vi "AlliGator Select Phasor Plot Data to Export Dialog.vi"(8 "error in (no error)":errorcluster) -> (0 "error out":errorcluster, 1 "OK?":bool caption="OK", 2 "Average Plot Data":bool, 3 "Phasor Plot Exported Data":T1)   [LabVIEW 2021, in "AlliGator Phasor Graph.lvlib"]
doc: "Dialog to select which phasor-related parameters to export as ASCII file."
uses:
  AlliGator Phasor Graph.lvlib
  AlliGator Phasor Plot Exported Data Selection.ctl
  GUI/GUI.lvlib
panel:
  in  "Deselect All":bool
  in  "Select All":bool
  in  "Show/Hide SDV":bool caption="Average Plot Data"
  in  "<tau> (amplitude-weighted) SDV":bool caption="<tau>"
  in  "phasor ratio (amplitude-weighted) SDV":bool caption="phasor ratio"
  in  "<tau> (intensity-weighted) SDV":bool caption="<tau>"
  in  "phasor ratio (intensity-weighted) SDV":bool caption="phasor ratio"
  in  "tau m SDV":bool caption="tau m"
  in  "tau phi SDV":bool caption="tau phi"
  in  "m SDV":bool caption="phi"
  in  "phi SDV":bool caption="m"
  in  "s SDV":bool caption="s"
  in  "g SDV":bool caption="g"
  in  "<tau> (amplitude-weighted)":bool caption="<tau>"
  in  "phasor ratio (amplitude-weighted)":bool caption="phasor ratio"
  in  "y":bool caption="s"
  in  "x":bool caption="g"
  in  "<tau> (intensity-weighted)":bool caption="<tau>"
  in  "phasor ratio (intensity-weighted)":bool caption="phasor ratio"
  in  "tau m":bool
  in  "tau phi":bool
  in  "m":bool caption="phi"
  in  "phi":bool caption="m"
  in  "s":bool
  in  "g":bool
  in  "Average Plot Data":bool
  in  "Cancel":bool
  in  "OK":bool caption="OK2"
  # "Select Phasor Plot Data to Export:"
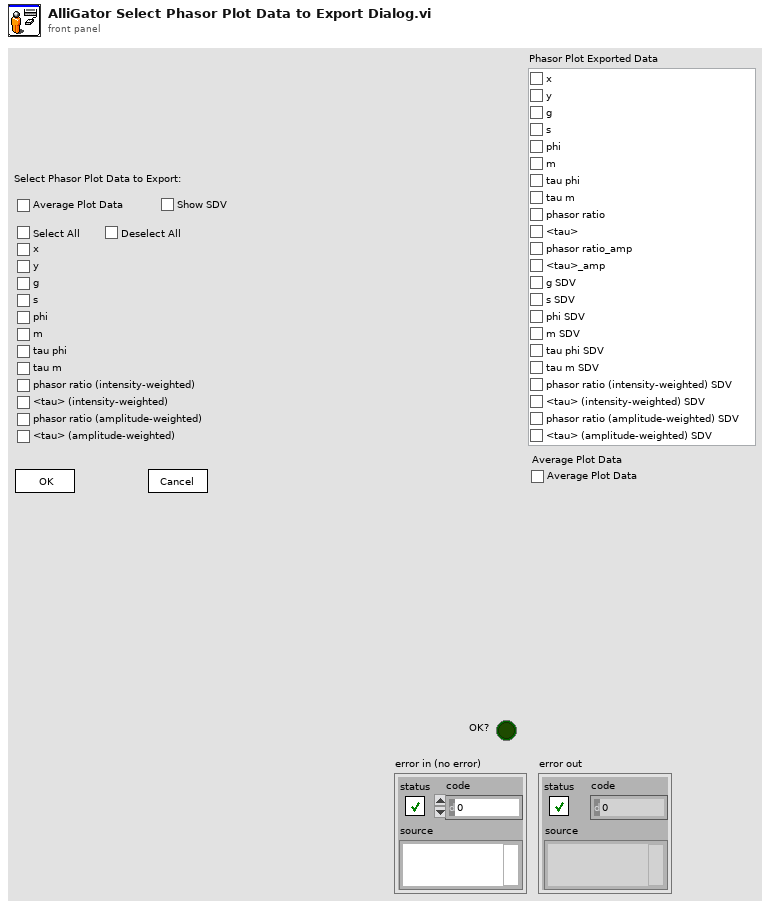
[diagram p1: front panel]
types:
  T1 = typedef "AlliGator Phasor Graph.lvlib/AlliGator Phasor Plot Exported Data Selection.ctl" = cluster{"x":bool, "y":bool, "g":bool, "s":bool, "phi":bool, "m":bool, "tau phi":bool, "tau m":bool, "phasor ratio (intensity-weighted)":bool, "<tau> (intensity-weighted)":bool, "phasor ratio (amplitude-weighted)":bool, "<tau> (amplitude-weighted)":bool, "g SDV":bool, "s SDV":bool, "phi SDV":bool, "m SDV":bool, "tau phi SDV":bool, "tau m SDV":bool, "phasor ratio (intensity-weighted) SDV":bool, "<tau> (intensity-weighted) SDV":bool, "phasor ratio (amplitude-weighted) SDV":bool, "<tau> (amplitude-weighted) SDV":bool}
  T2 = enum32{"Invalid", "Standard", "Closed", "Hidden", "Minimized", "Maximized"}
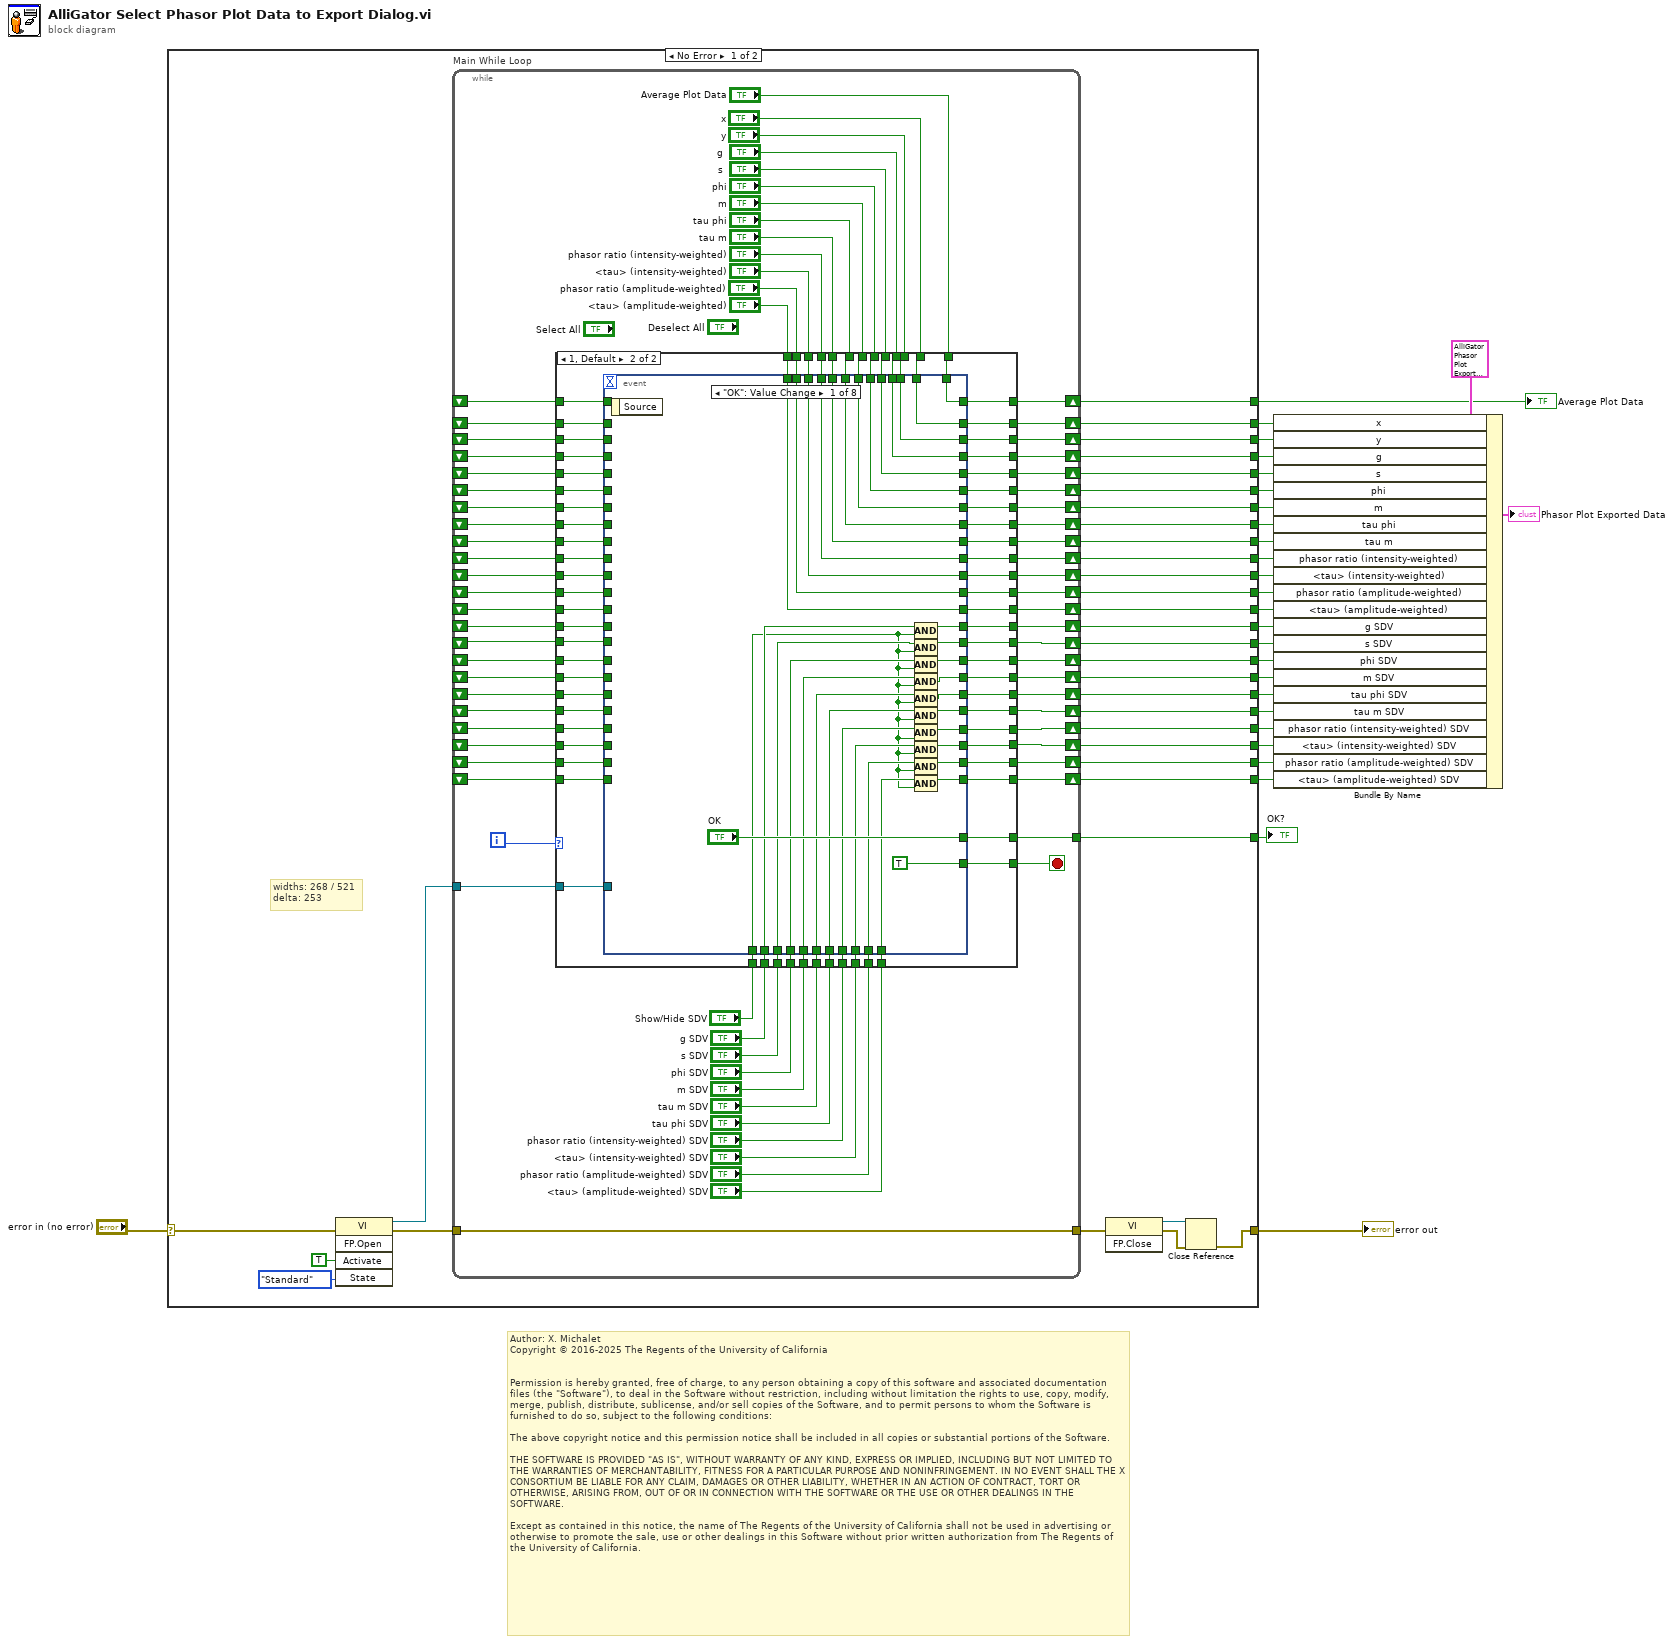
[diagram p0: block diagram]
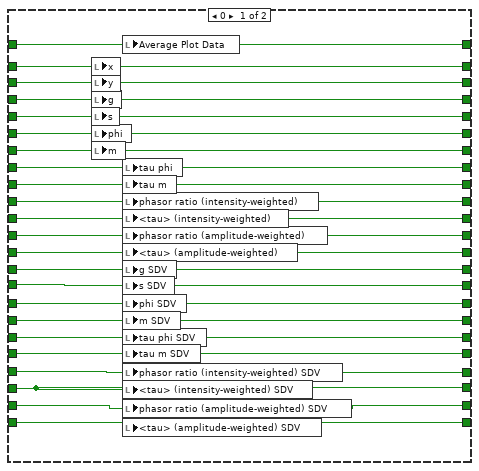
[diagram p2: hidden frame]
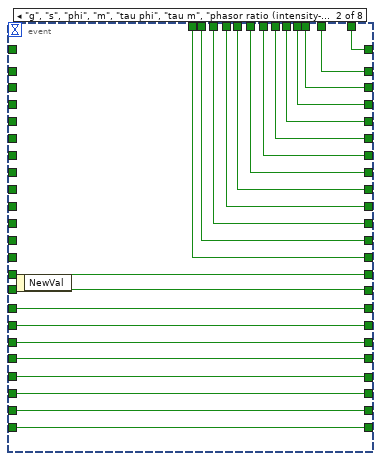
[diagram p3: hidden frame]
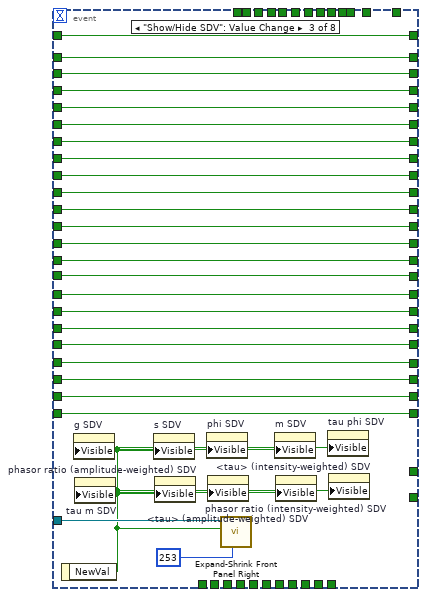
[diagram p4: hidden frame]
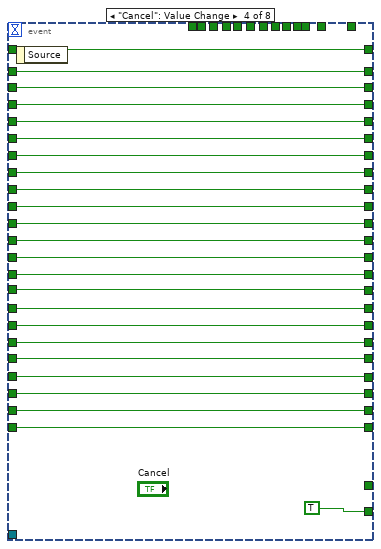
[diagram p5: hidden frame]
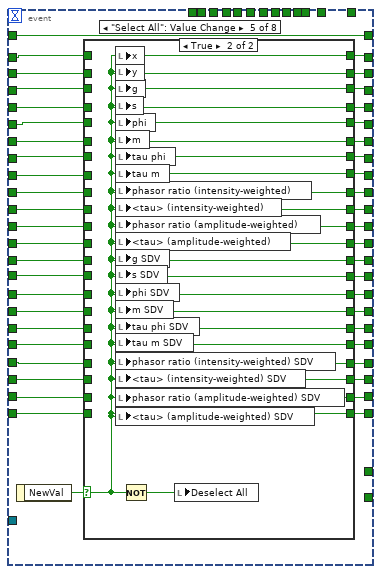
[diagram p6: hidden frame]
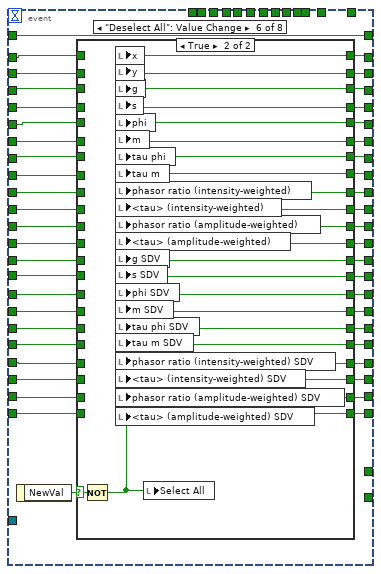
[diagram p8: hidden frame]
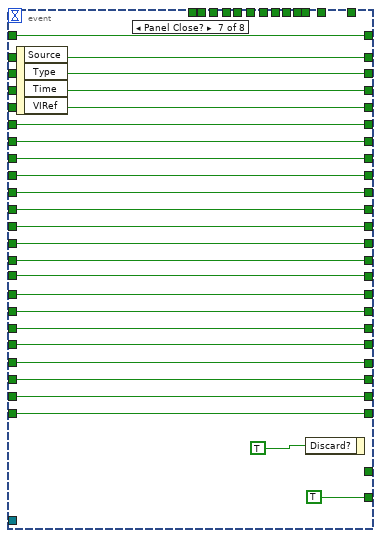
[diagram p10: hidden frame]
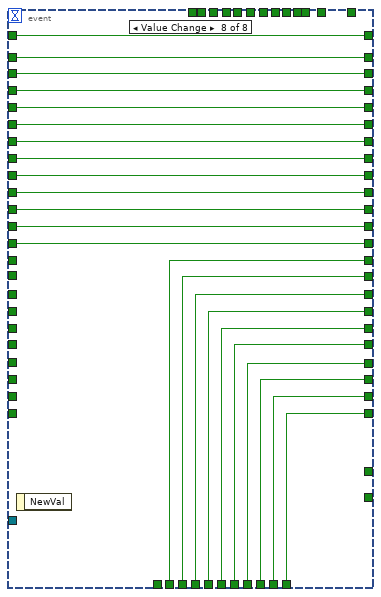
[diagram p11: hidden frame]
diagram:
  # "Author: X. Michalet\nCopyright © 2016-2025 The Regents of the University of California\n \n\nPermission is hereby granted, free of charge, to any person obtaining a copy of this software and associated documentation files (the \"Software\"), to deal in the Software without restriction, including without limitation the rights to use, copy, modify, merge, publish, distribute, sublicense, and/or sell copies of the Software, and to permit persons to whom the Software is furnished to do so, subject to the following conditions:\n\nThe above copyright notice and this permission notice shall be included in all copies or substantial portions of the Software.\n\nTHE SOFTWARE IS PROVIDED \"AS IS\", WITHOUT WARRANTY OF ANY KIND, EXPRESS OR IMPLIED, INCLUDING BUT NOT LIMITED TO THE WARRANTIES OF MERCHANTABILITY, FITNESS FOR A PARTICULAR PURPOSE AND NONINFRINGEMENT. IN NO EVENT SHALL THE X CONSORTIUM BE LIABLE FOR ANY CLAIM, DAMAGES OR OTHER LIABILITY, WHETHER IN AN ACTION OF CONTRACT, TORT OR OTHERWISE, ARISING FROM, OUT OF OR IN CONNECTION WITH THE SOFTWARE OR THE USE OR OTHER DEALINGS IN THE SOFTWARE.\n\nExcept as contained in this notice, the name of The Regents of the University of California shall not be used in advertising or otherwise to promote the sale, use or other dealings in this Software without prior written authorization from The Regents of the University of California."
  n1 = case shown="No Error" "error in (no error)" {
    selector: "error in (no error)" -> [w47 w530]
    tunnel: [w61 _] -> w27
    tunnel: [w60 _] -> w26
    tunnel: [w59 _] -> w25
    tunnel: [w58 _] -> w24
    tunnel: [w57 _] -> w23
    tunnel: [w56 _] -> w22
    tunnel: [w55 _] -> w21
    tunnel: [w54 _] -> w20
    tunnel: [w53 _] -> w19
    tunnel: [w52 _] -> w18
    tunnel: [w46 w530] -> w16
    tunnel: [w45 _] -> w14
    tunnel: [w44 _] -> w15
    tunnel: [w43 _] -> w12
    tunnel: [w42 _] -> w11
    tunnel: [w39 _] -> w10
    tunnel: [w38 _] -> w9
    tunnel: [w37 _] -> w8
    tunnel: [w36 _] -> w7
    tunnel: [w35 _] -> w6
    tunnel: [w34 _] -> w5
    tunnel: [w33 _] -> w4
    tunnel: [w32 _] -> w3
    tunnel: [w31 _] -> w2
    tunnel: [w30 _] -> w1
    frame No Error {
      # "widths: 268 / 521\ndelta: 253"
      n2 = invoke class="VI" method="FP.Open"(error in=w47, "Activate"=TRUE ("Activate?"), "State"=T2."Standard") -> (reference out=w29:refnum<vi>, error out=w41:errorcluster)  [unwired: 2 in, 3 out]
      n3 = while "Main While Loop" {
        shift-right: [w135] -> w60
        shift-left: _ -> [w117]
        shift-right: [w133] -> w59
        shift-left: _ -> [w116]
        shift-right: [w131] -> w58
        shift-left: _ -> [w115]
        shift-right: [w127] -> w57
        shift-left: _ -> [w114]
        shift-right: [w129] -> w56
        shift-left: _ -> [w113]
        shift-right: [w125] -> w55
        shift-left: _ -> [w112]
        shift-right: [w123] -> w54
        shift-left: _ -> [w111]
        shift-right: [w121] -> w53
        shift-left: _ -> [w110]
        shift-right: [w119] -> w52
        shift-left: _ -> [w109]
        tunnel: [w136] -> w61
        shift-right: [w104] -> w44
        shift-left: _ -> [w101]
        shift-right: [w106] -> w45
        shift-left: _ -> [w102]
        shift-right: [w99] -> w43
        shift-left: _ -> [w96]
        shift-right: [w97] -> w42
        shift-left: _ -> [w95]
        tunnel: w41 -> [w94]
        tunnel: [w94] -> w40
        shift-right: [w93] -> w39
        shift-left: _ -> [w73]
        shift-right: [w92] -> w38
        shift-left: _ -> [w72]
        shift-right: [w91] -> w37
        shift-left: _ -> [w71]
        shift-right: [w90] -> w36
        shift-left: _ -> [w70]
        shift-right: [w89] -> w35
        shift-left: _ -> [w69]
        shift-right: [w88] -> w34
        shift-left: _ -> [w68]
        shift-right: [w87] -> w33
        shift-left: _ -> [w67]
        shift-right: [w86] -> w32
        shift-left: _ -> [w66]
        shift-right: [w77] -> w31
        shift-left: _ -> [w65]
        shift-right: [w75] -> w30
        shift-left: _ -> [w64]
        tunnel: w29 -> [w63]
        i -> [w107]
        stop <- w108 stop-if-true
        n4 = case shown="1, Default" w107 {
          tunnel: [_ w232] -> w136
          tunnel: [w150 w231] -> w135
          tunnel: "Average Plot Data" -> [_ w230]
          tunnel: [w159 w229] -> w133
          tunnel: "g" -> [_ w228]
          tunnel: [w158 w227] -> w131
          tunnel: "s" -> [_ w226]
          tunnel: [w156 w225] -> w129
          tunnel: "m" -> [_ w224]
          tunnel: [w157 w223] -> w127
          tunnel: "phi" -> [_ w222]
          tunnel: [w155 w221] -> w125
          tunnel: "tau phi" -> [_ w220]
          tunnel: [w154 w219] -> w123
          tunnel: "tau m" -> [_ w218]
          tunnel: [w153 w217] -> w121
          tunnel: "phasor ratio (intensity-weighted)" -> [_ w216]
          tunnel: [w152 w215] -> w119
          tunnel: "<tau> (intensity-weighted)" -> [_ w214]
          tunnel: w117 -> [w150 w213]
          tunnel: w116 -> [w159 w212]
          tunnel: w115 -> [w158 w211]
          tunnel: w114 -> [w157 w210]
          tunnel: w113 -> [w156 w209]
          tunnel: w112 -> [w155 w208]
          tunnel: w111 -> [w154 w207]
          tunnel: w110 -> [w153 w206]
          tunnel: w109 -> [w152 w205]
          tunnel: [_ w204] -> w108
          tunnel: [w149 w203] -> w106
          tunnel: "y" -> [_ w202]
          tunnel: [w151 w201] -> w104
          tunnel: "x" -> [_ w200]
          tunnel: w102 -> [w149 w199]
          tunnel: w101 -> [w151 w198]
          tunnel: "phasor ratio (amplitude-weighted)" -> [_ w197]
          tunnel: [w148 w196] -> w99
          tunnel: "<tau> (amplitude-weighted)" -> [_ w195]
          tunnel: [w147 w194] -> w97
          tunnel: w96 -> [w148 w193]
          tunnel: w95 -> [w147 w192]
          tunnel: [w146 w191] -> w93
          tunnel: [w145 w189] -> w92
          tunnel: [w144 w187] -> w91
          tunnel: [w143 w185] -> w90
          tunnel: [w142 w183] -> w89
          tunnel: [w141 w181] -> w88
          tunnel: [w140 w179] -> w87
          tunnel: [w139 w177] -> w86
          tunnel: "g SDV" -> [_ w190]
          tunnel: "s SDV" -> [_ w188]
          tunnel: "phi SDV" -> [_ w186]
          tunnel: "m SDV" -> [_ w184]
          tunnel: "tau m SDV" -> [_ w182]
          tunnel: "tau phi SDV" -> [_ w180]
          tunnel: "phasor ratio (intensity-weighted) SDV" -> [_ w178]
          tunnel: "<tau> (intensity-weighted) SDV" -> [_ w176]
          tunnel: [w138 w175] -> w77
          tunnel: "phasor ratio (amplitude-weighted) SDV" -> [_ w174]
          tunnel: [w137 w173] -> w75
          tunnel: "<tau> (amplitude-weighted) SDV" -> [_ w172]
          tunnel: w73 -> [w146 w171]
          tunnel: w72 -> [w145 w170]
          tunnel: w71 -> [w144 w169]
          tunnel: w70 -> [w143 w168]
          tunnel: w69 -> [w142 w167]
          tunnel: w68 -> [w141 w166]
          tunnel: w67 -> [w140 w165]
          tunnel: w66 -> [w139 w164]
          tunnel: w65 -> [w138 w163]
          tunnel: w64 -> [w137 w162]
          tunnel: w63 -> [_ w161]
          tunnel: "Show/Hide SDV" -> [_ w160]
          frame 0 {
            n5 = local write "x"(w151) -> ()
            n6 = local write "y"(w150) -> ()
            n7 = local write "g"(w159) -> ()
            n8 = local write "s"(w158) -> ()
            n9 = local write "phi"(w157) -> ()
            n10 = local write "m"(w156) -> ()
            n11 = local write "Average Plot Data"(w149) -> ()
            n12 = local write "tau phi"(w155) -> ()
            n13 = local write "tau m"(w154) -> ()
            n14 = local write "phasor ratio (intensity-weighted)"(w153) -> ()
            n15 = local write "<tau> (intensity-weighted)"(w152) -> ()
            n16 = local write "phasor ratio (amplitude-weighted)"(w148) -> ()
            n17 = local write "<tau> (amplitude-weighted)"(w147) -> ()
            n18 = local write "g SDV"(w146) -> ()
            n19 = local write "s SDV"(w145) -> ()
            n20 = local write "phi SDV"(w144) -> ()
            n21 = local write "m SDV"(w143) -> ()
            n22 = local write "tau phi SDV"(w142) -> ()
            n23 = local write "tau m SDV"(w141) -> ()
            n24 = local write "phasor ratio (intensity-weighted) SDV"(w140) -> ()
            n25 = local write "<tau> (intensity-weighted) SDV"(w139) -> ()
            n26 = local write "phasor ratio (amplitude-weighted) SDV"(w138) -> ()
            n27 = local write "<tau> (amplitude-weighted) SDV"(w137) -> ()
          }
          frame 1, Default {
            n28 = event shown="[0] \"OK\": Value Change" {
              selector: _ -> [_ _ _ _ _ _ _ _]
              dyn-events: _ -> [_ _ _ _ _ _ _ _]
              timeout: _ -> [_ _ _ _ _ _ _ _]
              tunnel: ["OK" _ _ _ _ _ _ _] -> w232
              tunnel: [w257 w289 w317 w341 w384 w454 w506 w529] -> w231
              tunnel: w230 -> [w258 w291 _ _ _ _ _ _]
              tunnel: [w267 w288 w316 w340 w383 w453 w505 w528] -> w229
              tunnel: w228 -> [w267 w288 _ _ _ _ _ _]
              tunnel: [w266 w287 w315 w339 w382 w452 w504 w527] -> w227
              tunnel: w226 -> [w266 w287 _ _ _ _ _ _]
              tunnel: [w265 w285 w314 w337 w380 w450 w502 w525] -> w225
              tunnel: w224 -> [w265 w285 _ _ _ _ _ _]
              tunnel: [w264 w286 w313 w338 w381 w451 w503 w526] -> w223
              tunnel: w222 -> [w264 w286 _ _ _ _ _ _]
              tunnel: [w263 w284 w312 w336 w379 w449 w501 w524] -> w221
              tunnel: w220 -> [w263 w284 _ _ _ _ _ _]
              tunnel: [w262 w283 w311 w335 w378 w448 w500 w523] -> w219
              tunnel: w218 -> [w262 w283 _ _ _ _ _ _]
              tunnel: [w261 w282 w310 w334 w377 w447 w499 w522] -> w217
              tunnel: w216 -> [w261 w282 _ _ _ _ _ _]
              tunnel: [w260 w281 w309 w333 w376 w446 w498 w521] -> w215
              tunnel: w214 -> [w260 w281 _ _ _ _ _ _]
              tunnel: w213 -> [_ _ w317 w341 w362 w432 w506 w529]
              tunnel: w212 -> [_ _ w316 w340 w361 w431 w505 w528]
              tunnel: w211 -> [_ _ w315 w339 w360 w430 w504 w527]
              tunnel: w210 -> [_ _ w313 w338 w359 w429 w503 w526]
              tunnel: w209 -> [_ _ w314 w337 w358 w428 w502 w525]
              tunnel: w208 -> [_ _ w312 w336 w357 w427 w501 w524]
              tunnel: w207 -> [_ _ w311 w335 w356 w426 w500 w523]
              tunnel: w206 -> [_ _ w310 w334 w355 w425 w499 w522]
              tunnel: w205 -> [_ _ w309 w333 w354 w424 w498 w521]
              tunnel: [TRUE _ _ TRUE _ _ TRUE _] -> w204
              tunnel: [w258 w291 w308 w331 w387 w457 w495 w520] -> w203
              tunnel: w202 -> [w257 w289 _ _ _ _ _ _]
              tunnel: [w256 w290 w307 w330 w385 w455 w494 w519] -> w201
              tunnel: w200 -> [w256 w290 _ _ _ _ _ _]
              tunnel: w199 -> [_ _ w308 w331 w387 w457 w495 w520]
              tunnel: w198 -> [_ _ w307 w330 w363 w433 w494 w519]
              tunnel: w197 -> [w255 w280 _ _ _ _ _ _]
              tunnel: [w255 w280 w306 w329 w375 w445 w493 w518] -> w196
              tunnel: w195 -> [w254 w279 _ _ _ _ _ _]
              tunnel: [w254 w279 w305 w328 w374 w444 w492 w517] -> w194
              tunnel: w193 -> [_ _ w306 w329 w353 w423 w493 w518]
              tunnel: w192 -> [_ _ w305 w328 w352 w422 w492 w517]
              tunnel: [w252 w278 w304 w327 w373 w443 w491 w516] -> w191
              tunnel: w190 -> [w253 _ _ _ _ _ _ w516]
              tunnel: [w241 w277 w303 w326 w372 w442 w490 w515] -> w189
              tunnel: w188 -> [w251 _ _ _ _ _ _ w515]
              tunnel: [w240 w276 w302 w325 w371 w441 w489 w514] -> w187
              tunnel: w186 -> [w250 _ _ _ _ _ _ w514]
              tunnel: [w239 w275 w301 w324 w370 w440 w488 w513] -> w185
              tunnel: w184 -> [w249 _ _ _ _ _ _ w513]
              tunnel: [w238 w274 w300 w323 w369 w439 w487 w512] -> w183
              tunnel: w182 -> [w248 _ _ _ _ _ _ w512]
              tunnel: [w237 w273 w299 w322 w368 w438 w486 w511] -> w181
              tunnel: w180 -> [w247 _ _ _ _ _ _ w511]
              tunnel: [w236 w272 w298 w321 w367 w437 w485 w510] -> w179
              tunnel: w178 -> [w246 _ _ _ _ _ _ w510]
              tunnel: [w235 w271 w297 w320 w366 w436 w484 w509] -> w177
              tunnel: w176 -> [w245 _ _ _ _ _ _ w509]
              tunnel: [w234 w270 w296 w319 w365 w435 w483 w508] -> w175
              tunnel: w174 -> [w244 _ _ _ _ _ _ w508]
              tunnel: [w233 w269 w295 w318 w364 w434 w482 w507] -> w173
              tunnel: w172 -> [w243 _ _ _ _ _ _ w507]
              tunnel: w171 -> [_ w278 w304 w327 w351 w421 w491 _]
              tunnel: w170 -> [_ w277 w303 w326 w350 w420 w490 _]
              tunnel: w169 -> [_ w276 w302 w325 w349 w419 w489 _]
              tunnel: w168 -> [_ w275 w301 w324 w348 w418 w488 _]
              tunnel: w167 -> [_ w274 w300 w323 w347 w417 w487 _]
              tunnel: w166 -> [_ w273 w299 w322 w346 w416 w486 _]
              tunnel: w165 -> [_ w272 w298 w321 w345 w415 w485 _]
              tunnel: w164 -> [_ w271 w297 w320 w344 w414 w484 _]
              tunnel: w163 -> [_ w270 w296 w319 w343 w413 w483 _]
              tunnel: w162 -> [_ w269 w295 w318 w342 w412 w482 _]
              tunnel: w161 -> [_ _ w294 _ _ _ _ _]
              tunnel: w160 -> [w242 _ _ _ _ _ _ _]
              event "OK": Value Change {
                n29 = event-data() -> ()  [unwired: 1 in, 1 out]
                n30 = Compound Arithmetic op=AND(w253, w242) -> (w252:bool)
                n31 = Compound Arithmetic op=AND(w251, w242) -> (w241:bool)
                n32 = Compound Arithmetic op=AND(w250, w242) -> (w240:bool)
                n33 = Compound Arithmetic op=AND(w249, w242) -> (w239:bool)
                n34 = Compound Arithmetic op=AND(w248, w242) -> (w238:bool)
                n35 = Compound Arithmetic op=AND(w247, w242) -> (w237:bool)
                n36 = Compound Arithmetic op=AND(w246, w242) -> (w236:bool)
                n37 = Compound Arithmetic op=AND(w245, w242) -> (w235:bool)
                n38 = Compound Arithmetic op=AND(w244, w242) -> (w234:bool)
                n39 = Compound Arithmetic op=AND(w243, w242) -> (w233:bool)
              }
              event "g", "s", "phi", "m", "tau phi", "tau m", "phasor ratio (intensity-weighted)", "<tau> (intensity-weighted)", "x", "y", "Average Plot Data", "phasor ratio (amplitude-weighted)", "<tau> (amplitude-weighted)": Value Change {
                n40 = event-data() -> ()  [unwired: 1 in, 1 out]
              }
              event "Show/Hide SDV": Value Change {
                n41 = event-data() -> ("NewVal"=w292:bool)  [unwired: 1 in]
                n42 = property on="g SDV" class="Bool (strict)"("Visible"=w292) -> ()  [unwired: 2 in, 2 out]
                n43 = property on="tau m SDV" class="Bool (strict)"("Visible"=w292) -> ()  [unwired: 2 in, 2 out]
                n44 = property on="s SDV" class="Bool (strict)"("Visible"=w292) -> ()  [unwired: 2 in, 2 out]
                n45 = property on="phasor ratio (amplitude-weighted) SDV" class="Bool (strict)"("Visible"=w292) -> ()  [unwired: 2 in, 2 out]
                n46 = property on="phi SDV" class="Bool (strict)"("Visible"=w292) -> ()  [unwired: 2 in, 2 out]
                n47 = property on="<tau> (amplitude-weighted) SDV" class="Bool (strict)"("Visible"=w292) -> ()  [unwired: 2 in, 2 out]
                n48 = call "Expand-Shrink Front Panel Right.vi"("Side Panel Size"=253, "Expand(T)/Shrink"=w292, "VI Refnum"=w294) -> ()  [unwired: 8 in, 1 out]
                n49 = property on="m SDV" class="Bool (strict)"("Visible"=w292) -> ()  [unwired: 2 in, 2 out]
                n50 = property on="phasor ratio (intensity-weighted) SDV" class="Bool (strict)"("Visible"=w292) -> ()  [unwired: 2 in, 2 out]
                n51 = property on="tau phi SDV" class="Bool (strict)"("Visible"=w292) -> ()  [unwired: 2 in, 2 out]
                n52 = property on="<tau> (intensity-weighted) SDV" class="Bool (strict)"("Visible"=w292) -> ()  [unwired: 2 in, 2 out]
              }
              event "Cancel": Value Change {
                n53 = event-data() -> ()  [unwired: 1 in, 1 out]
              }
              event "Select All": Value Change {
                n54 = event-data() -> ("NewVal"=w386:bool)  [unwired: 1 in]
                n55 = case shown="True" w386 {
                  selector: w386 -> [_ w411]
                  tunnel: [w409 w411] -> w385
                  tunnel: [w408 w411] -> w384
                  tunnel: [w407 w411] -> w383
                  tunnel: [w406 w411] -> w382
                  tunnel: [w405 w411] -> w381
                  tunnel: [w404 w411] -> w380
                  tunnel: [w403 w411] -> w379
                  tunnel: [w402 w411] -> w378
                  tunnel: [w401 w411] -> w377
                  tunnel: [w400 w411] -> w376
                  tunnel: [w399 w411] -> w375
                  tunnel: [w398 w411] -> w374
                  tunnel: [w397 w411] -> w373
                  tunnel: [w396 w411] -> w372
                  tunnel: [w395 w411] -> w371
                  tunnel: [w394 w411] -> w370
                  tunnel: [w393 w411] -> w369
                  tunnel: [w392 w411] -> w368
                  tunnel: [w391 w411] -> w367
                  tunnel: [w390 w411] -> w366
                  tunnel: [w389 w411] -> w365
                  tunnel: [w388 w411] -> w364
                  tunnel: w363 -> [w409 _]
                  tunnel: w362 -> [w408 _]
                  tunnel: w361 -> [w407 _]
                  tunnel: w360 -> [w406 _]
                  tunnel: w359 -> [w405 _]
                  tunnel: w358 -> [w404 _]
                  tunnel: w357 -> [w403 _]
                  tunnel: w356 -> [w402 _]
                  tunnel: w355 -> [w401 _]
                  tunnel: w354 -> [w400 _]
                  tunnel: w353 -> [w399 _]
                  tunnel: w352 -> [w398 _]
                  tunnel: w351 -> [w397 _]
                  tunnel: w350 -> [w396 _]
                  tunnel: w349 -> [w395 _]
                  tunnel: w348 -> [w394 _]
                  tunnel: w347 -> [w393 _]
                  tunnel: w346 -> [w392 _]
                  tunnel: w345 -> [w391 _]
                  tunnel: w344 -> [w390 _]
                  tunnel: w343 -> [w389 _]
                  tunnel: w342 -> [w388 _]
                  frame False {
                  }
                  frame True {
                    n56 = local write "x"(w411) -> ()
                    n57 = local write "y"(w411) -> ()
                    n58 = local write "g"(w411) -> ()
                    n59 = local write "s"(w411) -> ()
                    n60 = local write "phi"(w411) -> ()
                    n61 = local write "m"(w411) -> ()
                    n62 = local write "tau phi"(w411) -> ()
                    n63 = local write "tau m"(w411) -> ()
                    n64 = local write "phasor ratio (intensity-weighted)"(w411) -> ()
                    n65 = local write "<tau> (intensity-weighted)"(w411) -> ()
                    n66 = local write "phasor ratio (amplitude-weighted)"(w411) -> ()
                    n67 = local write "<tau> (amplitude-weighted)"(w411) -> ()
                    n68 = local write "g SDV"(w411) -> ()
                    n69 = local write "s SDV"(w411) -> ()
                    n70 = local write "phi SDV"(w411) -> ()
                    n71 = local write "m SDV"(w411) -> ()
                    n72 = local write "tau phi SDV"(w411) -> ()
                    n73 = local write "tau m SDV"(w411) -> ()
                    n74 = local write "phasor ratio (intensity-weighted) SDV"(w411) -> ()
                    n75 = local write "<tau> (intensity-weighted) SDV"(w411) -> ()
                    n76 = local write "phasor ratio (amplitude-weighted) SDV"(w411) -> ()
                    n77 = local write "<tau> (amplitude-weighted) SDV"(w411) -> ()
                    n78 = Not(x=w411) -> (.not. x?=w410:bool)
                    n79 = local write "Deselect All"(w410) -> ()
                  }
                }
              }
              event "Deselect All": Value Change {
                n80 = event-data() -> ("NewVal"=w456:bool)  [unwired: 1 in]
                n81 = case shown="True" w456 {
                  selector: w456 -> [_ w481]
                  tunnel: [w479 w480] -> w455
                  tunnel: [w478 w480] -> w454
                  tunnel: [w477 w480] -> w453
                  tunnel: [w476 w480] -> w452
                  tunnel: [w475 w480] -> w451
                  tunnel: [w474 w480] -> w450
                  tunnel: [w473 w480] -> w449
                  tunnel: [w472 w480] -> w448
                  tunnel: [w471 w480] -> w447
                  tunnel: [w470 w480] -> w446
                  tunnel: [w469 w480] -> w445
                  tunnel: [w468 w480] -> w444
                  tunnel: [w467 w480] -> w443
                  tunnel: [w466 w480] -> w442
                  tunnel: [w465 w480] -> w441
                  tunnel: [w464 w480] -> w440
                  tunnel: [w463 w480] -> w439
                  tunnel: [w462 w480] -> w438
                  tunnel: [w461 w480] -> w437
                  tunnel: [w460 w480] -> w436
                  tunnel: [w459 w480] -> w435
                  tunnel: [w458 w480] -> w434
                  tunnel: w433 -> [w479 _]
                  tunnel: w432 -> [w478 _]
                  tunnel: w431 -> [w477 _]
                  tunnel: w430 -> [w476 _]
                  tunnel: w429 -> [w475 _]
                  tunnel: w428 -> [w474 _]
                  tunnel: w427 -> [w473 _]
                  tunnel: w426 -> [w472 _]
                  tunnel: w425 -> [w471 _]
                  tunnel: w424 -> [w470 _]
                  tunnel: w423 -> [w469 _]
                  tunnel: w422 -> [w468 _]
                  tunnel: w421 -> [w467 _]
                  tunnel: w420 -> [w466 _]
                  tunnel: w419 -> [w465 _]
                  tunnel: w418 -> [w464 _]
                  tunnel: w417 -> [w463 _]
                  tunnel: w416 -> [w462 _]
                  tunnel: w415 -> [w461 _]
                  tunnel: w414 -> [w460 _]
                  tunnel: w413 -> [w459 _]
                  tunnel: w412 -> [w458 _]
                  frame False {
                  }
                  frame True {
                    n82 = Not(x=w481) -> (.not. x?=w480:bool)
                    n83 = local write "x"(w480) -> ()
                    n84 = local write "y"(w480) -> ()
                    n85 = local write "g"(w480) -> ()
                    n86 = local write "s"(w480) -> ()
                    n87 = local write "phi"(w480) -> ()
                    n88 = local write "m"(w480) -> ()
                    n89 = local write "tau phi"(w480) -> ()
                    n90 = local write "tau m"(w480) -> ()
                    n91 = local write "phasor ratio (intensity-weighted)"(w480) -> ()
                    n92 = local write "<tau> (intensity-weighted)"(w480) -> ()
                    n93 = local write "phasor ratio (amplitude-weighted)"(w480) -> ()
                    n94 = local write "<tau> (amplitude-weighted)"(w480) -> ()
                    n95 = local write "g SDV"(w480) -> ()
                    n96 = local write "s SDV"(w480) -> ()
                    n97 = local write "phi SDV"(w480) -> ()
                    n98 = local write "m SDV"(w480) -> ()
                    n99 = local write "tau phi SDV"(w480) -> ()
                    n100 = local write "tau m SDV"(w480) -> ()
                    n101 = local write "phasor ratio (intensity-weighted) SDV"(w480) -> ()
                    n102 = local write "<tau> (intensity-weighted) SDV"(w480) -> ()
                    n103 = local write "phasor ratio (amplitude-weighted) SDV"(w480) -> ()
                    n104 = local write "<tau> (amplitude-weighted) SDV"(w480) -> ()
                    n105 = local write "Select All"(w480) -> ()
                  }
                }
              }
              event Panel Close? {
                n106 = event-data() -> ()  [unwired: 1 in, 4 out]
                n107 = event-data("Discard?"=TRUE) -> ()  [unwired: 1 in, 1 out]
              }
              event Value Change {
                n108 = event-data() -> ()  [unwired: 1 in, 1 out]
              }
            }
          }
        }
      }
      n109 = invoke class="VI" method="FP.Close"(error in=w40) -> (reference out=w49:refnum<vi>, error out=w48:errorcluster)  [unwired: 2 in, 1 out]
      n110 = Close Reference(reference=w49, error in (no error)=w48) -> (error out=w46:errorcluster)
    }
    frame Error {
    }
  }
  "OK?" <- w27
  "error out" <- w16
  "Average Plot Data" <- w14
  n111 = Bundle By Name(cluster=T1 {"x"=FALSE, "y"=FALSE, "g"=FALSE, "s"=FALSE, "phi"=FALSE, "m"=FALSE, "tau phi"=FALSE, "tau m"=FALSE, "phasor ratio (intensity-weighted)"=FALSE, "<tau> (intensity-weighted)"=FALSE, "phasor ratio (amplitude-weighted)"=FALSE, "<tau> (amplitude-weighted)"=FALSE, "g SDV"=FALSE, "s SDV"=FALSE, "phi SDV"=FALSE, "m SDV"=FALSE, "tau phi SDV"=FALSE, "tau m SDV"=FALSE, "phasor ratio (intensity-weighted) SDV"=FALSE, "<tau> (intensity-weighted) SDV"=FALSE, "phasor ratio (amplitude-weighted) SDV"=FALSE, "<tau> (amplitude-weighted) SDV"=FALSE} ("Phasor Plot Exported Data"), "x"=w15, "y"=w26, "g"=w25, "s"=w24, "phi"=w23, "m"=w22, "tau phi"=w21, "tau m"=w20, "phasor ratio (intensity-weighted)"=w19, "<tau> (intensity-weighted)"=w18, "phasor ratio (amplitude-weighted)"=w12, "<tau> (amplitude-weighted)"=w11, "g SDV"=w10, "s SDV"=w9, "phi SDV"=w8, "m SDV"=w7, "tau phi SDV"=w6, "tau m SDV"=w5, "phasor ratio (intensity-weighted) SDV"=w4, "<tau> (intensity-weighted) SDV"=w3, "phasor ratio (amplitude-weighted) SDV"=w2, "<tau> (amplitude-weighted) SDV"=w1) -> (→"Phasor Plot Exported Data":T1)
